vi "showUI.vi"(8 "error in (no error)":errorcluster, 11 "Inst.Transport in":refnum<class "Inst.Transport.lvclass">) -> (0 "error out":errorcluster, 3 "Inst.Transport out":refnum<class "Inst.Transport.lvclass">)   [LabVIEW 2019, in "Inst.Transport.lvclass"]
uses:
  Inst.Transport.lvclass
  C:/Program Files (x86)/National Instruments/LabVIEW 2019/user.lib/LevyLab/Instrument Framework/Instrument/Instrument.lvclass
  Typedefs/Inst.Transport.ProtectedCommands--Enum.ctl
  <userlib>/LevyLab/Instrument Framework/Instrument/Typedefs/Client Type--Enum.ctl
  <userlib>/LevyLab/Instrument Framework/Instrument/Instrument.lvclass/Instrument.ctl
  <userlib>/LevyLab/Instrument Framework/Instrument/Instrument.lvclass
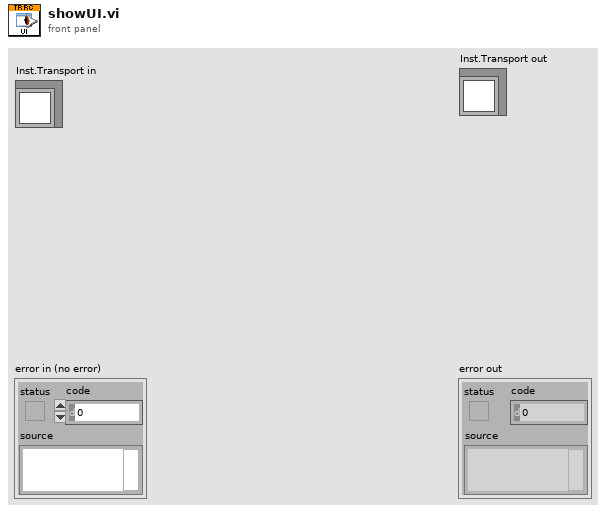
[diagram p1: front panel]
types:
  T1 = typedef "Instrument.lvlib/Instrument.lvclass/Client Type--Enum.ctl" = enum16{"Remote", "Local"}
  T2 = typedef "Inst.Transport.lvclass/Inst.Transport.ProtectedCommands--Enum.ctl" = enum16{"setStatus", "showUI", "hideUI"}
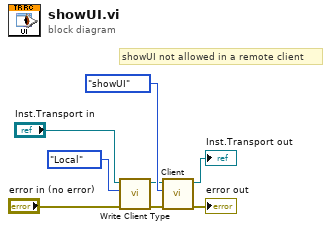
[diagram p0: block diagram]
diagram:
  # "showUI not allowed in a remote client"
  n1 = call <userlib>:"Write Client Type.vi"("error in (no error)"="error in (no error)", "Client Type [Remote]"=Client_Type--Enum."Local", "Instrument in"="Inst.Transport in") -> ("error out"=w1:errorcluster, "Instrument out"=w2:refnum<class "Inst.Transport.lvclass">)  [unwired: 7 in]
  n2 = call-dynamic "Client.vi"("error in (no error)"=w1, "Command in"=Inst.Transport.ProtectedCommands--Enum."showUI" ("ProtectedCommands"), "Instrument in"=w2) -> ("error out"=→"error out":errorcluster, "Instrument out"=→"Inst.Transport out":refnum<class "Inst.Transport.lvclass">)  [unwired: 5 in, 2 out]
